vi "fix dynamic mapping.vi"(8 "error in":errorcluster, 10 "DecideProjectFeatures in":refnum<class "TagBusConfigurablePluginDecideFeatures.lvclass">, 11 "User Project in":refnum<vi>) -> (0 "error out":errorcluster, 3 "User Project out":refnum<vi>)   [LabVIEW 2013, in "TagBusConfigurablePluginDecideFeatures.lvclass"]
uses:
  TagBusConfigurablePluginDecideFeatures.lvclass
  TagBusConfigurablePluginDecideFeatures.lvclass/TagBusConfigurablePluginDecideFeatures.ctl
  <vilib>/Utility/traverseref.llb/TRef TravTarget.ctl
  Read perform dynamic mapping.vi
  Read perform dynamic reads.vi
  Read perform dynamic writes.vi
  <vilib>/Utility/traverseref.llb/VI Scripting - Traverse.lvlib
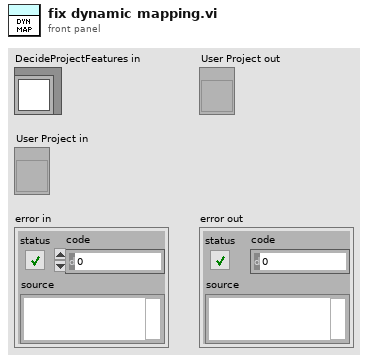
[diagram p1: front panel]
types:
  T1 = typedef "TRef TravTarget.ctl" = enum16{"FP", "BD", "Other"}
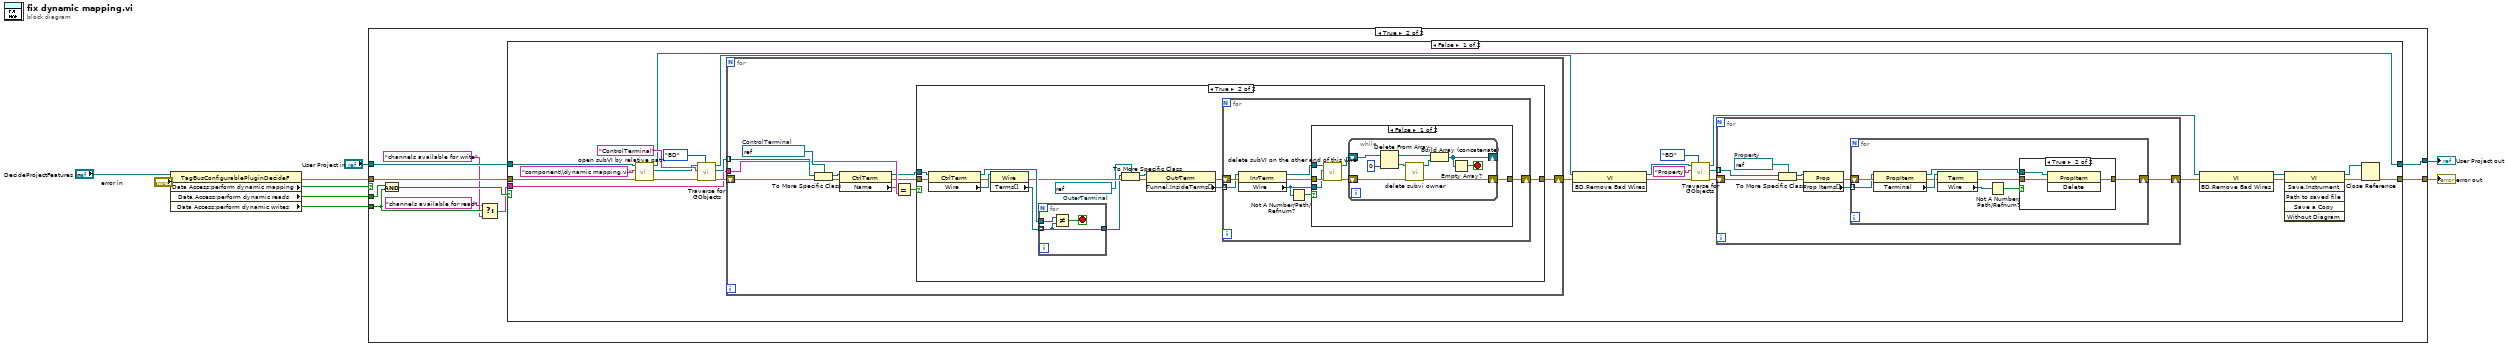
[diagram p0: block diagram]
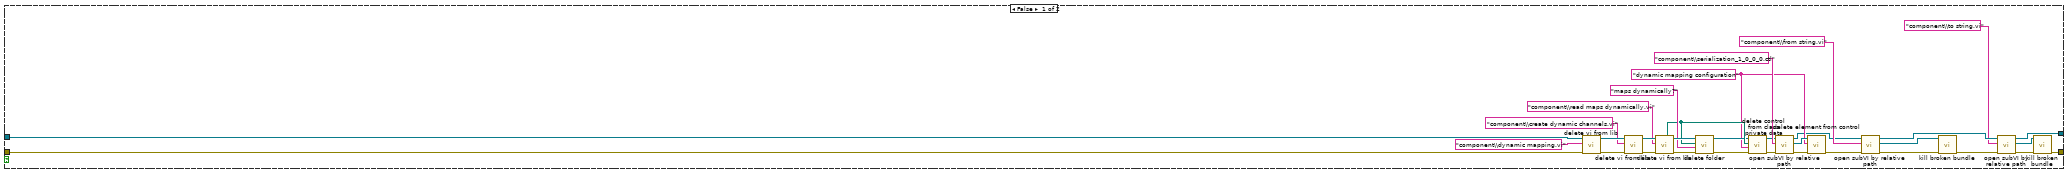
[diagram p2: hidden frame]
diagram:
  n1 = property class="TagBusConfigurablePluginDecideF"(reference="DecideProjectFeatures in", error in="error in") -> (error out=w4:errorcluster, "Data Access:perform dynamic mapping"=w7:bool, "Data Access:perform dynamic reads"=w2:bool, "Data Access:perform dynamic writes"=w1:bool)  [unwired: 1 out]
  n2 = case shown="True" w7 {
    tunnel: "User Project in" -> [w41 w47]
    tunnel: [w10 w48] -> w5
    tunnel: w4 -> [w40 w49]
    tunnel: [w11 w50] -> w3
    tunnel: w2 -> [_ w52]
    tunnel: w1 -> [_ w46]
    frame False {
      w22 = "dynamic mapping configuration" ("folder")
      n3 = call "delete vi from lib.vi"("error in"=w40, "relative path"="component\\dynamic mapping.vi", "Project in"=w41) -> ("error out"=w38:errorcluster, "Project out"=w39:refnum<vi>)  [unwired: 6 in, 1 out]
      n4 = call "delete vi from lib.vi"("error in"=w38, "relative path"="component\\create dynamic channels.vi", "Project in"=w39) -> ("error out"=w35:errorcluster, "Project out"=w36:refnum<vi>)  [unwired: 6 in, 1 out]
      n5 = call "delete vi from lib.vi"("error in"=w35, "relative path"="component\\read maps dynamically.vi", "Project in"=w36) -> ("error out"=w32:errorcluster, "Project out"=w33:refnum<vi>, "lib path"=w30:path)  [unwired: 6 in]
      n6 = call "delete folder.vi"("error in"=w32, "folder"="maps dynamically?", "lib path"=w30, "Project in"=w33) -> ("error out"=w28:errorcluster, "Project out"=w29:refnum<vi>)  [unwired: 6 in]
      n7 = call "delete control from class private data.vi"("error in"=w28, "control label"=w22, "path"=w30, "Project in"=w29) -> ("error out"=w23:errorcluster, "Project out"=w24:refnum<vi>)  [unwired: 6 in]
      n8 = call "open subVI by relative path.vi"("error in"=w23, "relative path"="component\\serialization_1_0_0_0.ctl", "Project in"=w24) -> ("error out"=w26:errorcluster, "vi reference"=w27:refnum<vi>, "Project out"=w13:refnum<vi>)  [unwired: 6 in]
      n9 = call "delete element from control.vi"("error in"=w26, "control label"=w22, "VI in"=w27) -> ("error out"=w12:errorcluster)  [unwired: 8 in]
      n10 = call "open subVI by relative path.vi"("error in"=w12, "relative path"="component\\from string.vi", "Project in"=w13) -> ("error out"=w16:errorcluster, "vi reference"=w18:refnum<vi>, "Project out"=w21:refnum<vi>)  [unwired: 6 in]
      n11 = call "kill broken bundle.vi"("error in"=w16, "VI in"=w18) -> ("error out"=w17:errorcluster)  [unwired: 9 in]
      n12 = call "open subVI by relative path.vi"("error in"=w17, "relative path"="component\\to string.vi", "Project in"=w21) -> ("error out"=w14:errorcluster, "vi reference"=w15:refnum<vi>, "Project out"=w10:refnum<vi>)  [unwired: 6 in]
      n13 = call "kill broken bundle.vi"("error in"=w14, "VI in"=w15) -> ("error out"=w11:errorcluster)  [unwired: 9 in]
    }
    frame True {
      n14 = Compound Arithmetic op=AND(w52, w46) -> (w51:bool)
      n15 = Select(t="channels available for read", s=w46, f="channels available for write") -> (s? t:f=w43:string)
      n16 = case shown="False" w51 {
        tunnel: [w78 w153] -> w50
        tunnel: w49 -> [w65 w153]
        tunnel: [w67 w152] -> w48
        tunnel: w47 -> [w64 w152]
        tunnel: w43 -> [w72 _]
        frame False {
          n17 = call "open subVI by relative path.vi"("error in"=w65, "relative path"="component\\dynamic mapping.vi", "Project in"=w64) -> ("error out"=w66:errorcluster, "vi reference"=w68:refnum<vi>, "Project out"=w67:refnum<vi>)  [unwired: 6 in]
          n18 = call <vilib>:"Traverse for GObjects.vi"("Traverse Target"=TRef_TravTarget."BD", "error in (no error)"=w66, "Class Name"="ControlTerminal", "VI Refnum"=w68) -> ("error out"=w75:errorcluster, "References"=w73:refnum<vi>[], "dup VI Refnum"=w71:refnum<vi>)  [unwired: 4 in, 1 out]
          n19 = for {
            shift-right: [w101] -> w74
            shift-left: w75 -> [w110]
            tunnel: w73 -> [w108] mode=indexing
            tunnel: w72 -> [w105]
            w109 = refnum<vi> refnum  # ControlTerminal
            n20 = To More Specific Class(target class=w109, reference=w108, error in=w110) -> (specific class reference=w107:refnum<vi>, error out=w106:errorcluster)
            n21 = property class="CtrlTerm"(reference=w107, error in=w106) -> (reference out=w100:refnum<vi>, error out=w102:errorcluster, "Name"=w104:string)
            n22 = Equal?(x=w104, y=w105) -> (x = y?=w103:bool)
            n23 = case shown="True" w103 {
              tunnel: w102 -> [w111 w124]
              tunnel: [w111 w112] -> w101
              tunnel: w100 -> [_ w125]
              frame False {
              }
              frame True {
                w117 = refnum<vi> refnum  # OuterTerminal
                n24 = property class="CtrlTerm"(reference=w125, error in=w124) -> (reference out=w120:refnum<vi>, error out=w122:errorcluster, "Wire"=w123:refnum<vi>)
                n25 = property class="Wire"(reference=w123, error in=w122) -> (error out=w119:errorcluster, "Terms[]"=w121:refnum<vi>[])  [unwired: 1 out]
                n26 = for {
                  tunnel: w121 -> [w149] mode=indexing
                  tunnel: w120 -> [w151]
                  tunnel: [w149] -> w118
                  stop <- w150 stop-if-true
                  n27 = Not Equal?(x=w151, y=w149) -> (x != y?=w150:bool)
                }
                n28 = To More Specific Class(target class=w117, reference=w118, error in=w119) -> (specific class reference=w116:refnum<vi>, error out=w115:errorcluster)
                n29 = property class="OutrTerm"(reference=w116, error in=w115) -> (error out=w114:errorcluster, "Tunnel.InsideTerms[]"=w113:refnum<vi>[])  [unwired: 1 out]
                n30 = for {
                  shift-right: [w129] -> w112
                  shift-left: w114 -> [w132]
                  tunnel: w113 -> [w131] mode=indexing
                  n31 = property class="InrTerm"(reference=w131, error in=w132) -> (reference out=w126:refnum<vi>, error out=w128:errorcluster, "Wire"=w127:refnum<vi>)
                  n32 = Not A Number/Path/Refnum?(number/path/refnum=w127) -> (NaN/Path/Refnum?=w130:bool)
                  n33 = case shown="False" w130 {
                    tunnel: [w133 w148] -> w129
                    tunnel: w128 -> [w138 w148]
                    tunnel: w127 -> [w137 _]
                    tunnel: w126 -> [w136 _]
                    frame False {
                      n34 = call "delete subVI on the other end of this wire.vi"("error in"=w138, "Wire"=w137, "source term"=w136) -> ("error out"=w135:errorcluster, "connected terminals"=w134:refnum<vi>[])  [unwired: 7 in]
                      n35 = while {
                        shift-right: [w141] -> w133
                        shift-left: w135 -> [w147]
                        shift-right: [w140] -> _
                        shift-left: w134 -> [w146]
                        stop <- w139 stop-if-true
                        n36 = Delete From Array(array=w146, index=0) -> (deleted portion=w145:refnum<vi>, array with subset deleted=w143:refnum<vi>[])  [unwired: 1 in]
                        n37 = call "delete subvi owner.vi"("error in"=w147, "Terminal in"=w145) -> ("error out"=w141:errorcluster, "other terminals"=w142:refnum<vi>[])  [unwired: 8 in]
                        n38 = Build Array (concatenate)(w143, w142) -> (w140:refnum<vi>[])
                        n39 = Empty Array?(array=w140) -> (empty?=w139:bool)
                      }
                    }
                    frame True {
                    }
                  }
                }
              }
            }
          }
          n40 = invoke class="VI" method="BD.Remove Bad Wires"(reference=w71, error in=w74) -> (reference out=w55:refnum<vi>, error out=w56:errorcluster)  [unwired: 1 in, 1 out]
          n41 = call <vilib>:"Traverse for GObjects.vi"("Traverse Target"=TRef_TravTarget."BD", "error in (no error)"=w56, "Class Name"="Property", "VI Refnum"=w55) -> ("error out"=w61:errorcluster, "References"=w59:refnum<vi>[], "dup VI Refnum"=w57:refnum<vi>)  [unwired: 4 in, 1 out]
          n42 = for {
            shift-right: [w79] -> w60
            shift-left: w61 -> [w86]
            tunnel: w59 -> [w85] mode=indexing
            w84 = refnum<vi> refnum  # Property
            n43 = To More Specific Class(target class=w84, reference=w85, error in=w86) -> (specific class reference=w83:refnum<vi>, error out=w82:errorcluster)
            n44 = property class="Prop"(reference=w83, error in=w82) -> (error out=w81:errorcluster, "Prop Items[]"=w80:refnum<vi>[])  [unwired: 1 out]
            n45 = for {
              shift-right: [w87] -> w79
              shift-left: w81 -> [w95]
              tunnel: w80 -> [w94] mode=indexing
              n46 = property class="PropItem"(reference=w94, error in=w95) -> (reference out=w88:refnum<vi>, error out=w91:errorcluster, "Terminal"=w93:refnum<vi>)
              n47 = property class="Term"(reference=w93, error in=w91) -> (error out=w89:errorcluster, "Wire"=w92:refnum<vi>)  [unwired: 1 out]
              n48 = Not A Number/Path/Refnum?(number/path/refnum=w92) -> (NaN/Path/Refnum?=w90:bool)
              n49 = case shown="True" w90 {
                tunnel: w89 -> [w96 w99]
                tunnel: w88 -> [_ w98]
                tunnel: [w96 w97] -> w87
                frame False {
                }
                frame True {
                  n50 = invoke class="PropItem" method="Delete"(reference=w98, error in=w99) -> (error out=w97:errorcluster)  [unwired: 1 in, 2 out]
                }
              }
            }
          }
          n51 = invoke class="VI" method="BD.Remove Bad Wires"(reference=w57, error in=w60) -> (reference out=w53:refnum<vi>, error out=w54:errorcluster)  [unwired: 1 in, 1 out]
          n52 = invoke class="VI" method="Save.Instrument"(reference=w53, error in=w54) -> (reference out=w69:refnum<vi>, error out=w70:errorcluster)  [unwired: 4 in, 4 out]
          n53 = Close Reference(reference=w69, error in (no error)=w70) -> (error out=w78:errorcluster)
        }
        frame True {
          # "as written"
        }
      }
    }
  }
  "error out" <- w3
  "User Project out" <- w5
